vi "Example Callback.vi"() -> ()   [LabVIEW 2010]
uses:
  C:/tf/play/labview/Tinkerforge.dll
panel:
  in  "stop":bool
  in  "uid":string="6dKCNw"
  in  "port":i32=4223
  in  "host":string="localhost"
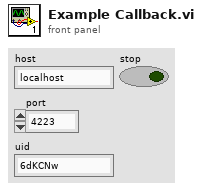
[diagram p1: front panel]
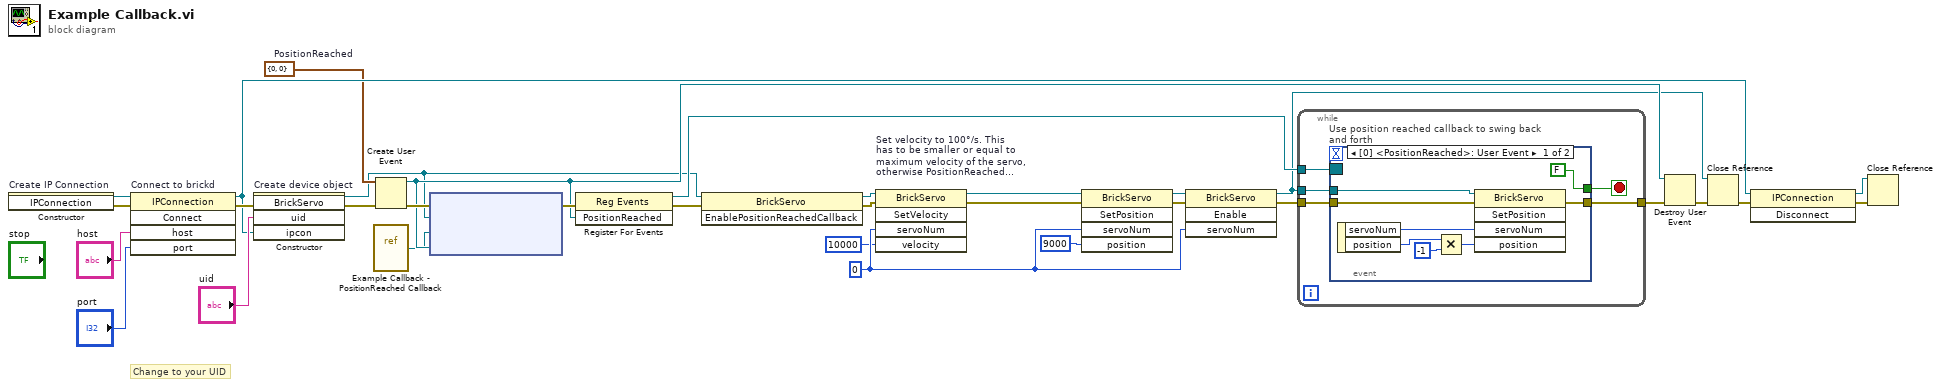
[diagram p0: block diagram]
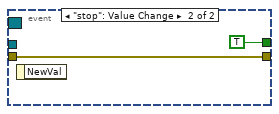
[diagram p2: hidden frame]
diagram:
  w9 = u8 0 ("servoNum")
  w17 = cluster{"servoNum":u8, "position":i16} {"servoNum"=0, "position"=0}  # PositionReached
  # "Change to your UID"
  n1 = constructor on="Create IP Connection" class="IPConnection"() -> (reference out=w32:refnum<k24>, error out=w1:errorcluster)  [unwired: 3 in, 1 out]
  n2 = invoke on="Connect to brickd" class="IPConnection" method="Connect"(reference=w32, error in=w1, "host"="host", "port"="port") -> (reference out=w25:refnum<k24>, error out=w28:errorcluster)  [unwired: 1 in, 3 out]
  n3 = constructor on="Create device object" class="BrickServo"(error in=w28, "uid"="uid", "ipcon"=w25) -> (reference out=w3:refnum<k24>, error out=w16:errorcluster)  [unwired: 2 in, 3 out]
  n4 = vi-ref "Example Callback - PositionReached Callback.vi"() -> ("vi reference"=w6:refnum<vi>)
  n5 = Create User Event(user event datatype=w17, error in=w16) -> (user event=w19:refnum<user-event>, error out=w23:errorcluster)
  n6 = node ("Register Event Callback")(w23, w3, w6, w19) -> (w22:errorcluster)  [unwired: 1 in, 1 out]
  n7 = register-events(error in=w22, w19) -> (reference out=w21:refnum<event-registration>, error out=w5:errorcluster)  [unwired: 1 in]
  n8 = invoke class="BrickServo" method="EnablePositionReachedCallback"(reference=w3, error in=w5) -> (reference out=w2:refnum<k24>, error out=w4:errorcluster)  [unwired: 1 in, 1 out]
  n9 = invoke on="Set velocity to 100°/s. This\nhas to be smaller or equal to\nmaximum velocity of the servo,\notherwise PositionReached\nwill be called too early" class="BrickServo" method="SetVelocity"(reference=w2, error in=w4, "servoNum"=w9, "velocity"=10000) -> (reference out=w15:refnum<k24>, error out=w14:errorcluster)  [unwired: 1 in, 3 out]
  n10 = invoke class="BrickServo" method="SetPosition"(reference=w15, error in=w14, "servoNum"=w9, "position"=i16 9000) -> (reference out=w10:refnum<k24>, error out=w13:errorcluster)  [unwired: 1 in, 3 out]
  n11 = invoke class="BrickServo" method="Enable"(reference=w10, error in=w13, "servoNum"=w9) -> (reference out=w11:refnum<k24>, error out=w12:errorcluster)  [unwired: 1 in, 2 out]
  n12 = while {
    tunnel: w21 -> [w37]
    tunnel: [w36] -> w20
    tunnel: w12 -> [w35]
    tunnel: w11 -> [w34]
    stop <- w33 stop-if-true
    n13 = event "Use position reached callback to swing back and forth" shown="[0] <PositionReached>: User Event" {
      selector: w37 -> [_ _]
      dyn-events: _ -> [_ _]
      timeout: _ -> [_ _]
      tunnel: [w45 w46] -> w36
      tunnel: w35 -> [w43 w46]
      tunnel: w34 -> [w42 _]
      tunnel: [FALSE TRUE] -> w33
      event User Event {
        n14 = event-data() -> ("servoNum"=w41:u8, "position"=w40:i16)  [unwired: 1 in]
        n15 = Multiply(x=w40, y=i16 -1) -> (x*y=w39:i16)
        n16 = invoke class="BrickServo" method="SetPosition"(reference=w42, error in=w43, "servoNum"=w41, "position"=w39) -> (error out=w45:errorcluster)  [unwired: 1 in, 4 out]
      }
      event "stop": Value Change {
        n17 = event-data() -> ()  [unwired: 1 in, 1 out]
      }
    }
  }
  n18 = Destroy User Event(user event=w19, error in=w20) -> (error out=w18:errorcluster)
  n19 = Close Reference(reference=w11, error in (no error)=w18) -> (error out=w27:errorcluster)
  n20 = invoke class="IPConnection" method="Disconnect"(reference=w25, error in=w27) -> (reference out=w24:refnum<k24>, error out=w26:errorcluster)  [unwired: 1 in, 1 out]
  n21 = Close Reference(reference=w24, error in (no error)=w26) -> ()  [unwired: 1 out]
